vi "4155C Config I Stress v2.0.vi"(3 "Stress I - Drain/Gate":u32(ring)=1 items=["SMU1  ", "SMU2  ", "SMU3  ", "SMU4  ", "SMU5  ", "SMU6  "], 4 "Stress I - Source/Common":u32(ring) items=["SMU1  ", "SMU2  ", "SMU3  ", "SMU4  ", "SMU5  ", "SMU6  "], 5 "Display on/off":bool, 6 "error in (no error)":errorcluster, 7 "VDG compliance":dbl min=0.0 max=100000000000.0 format="%.15e", 8 "IDG":dbl min=0.0 max=100000000000.0 format="%.15e", 9 "VISA session":refnum<visa-resource-name>) -> (0 "error out":errorcluster, 2 "dup VISA resource name":refnum<visa-resource-name>)   [LabVIEW 2016]
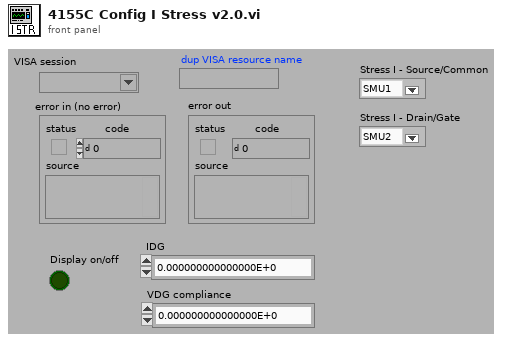
[diagram p1: front panel]
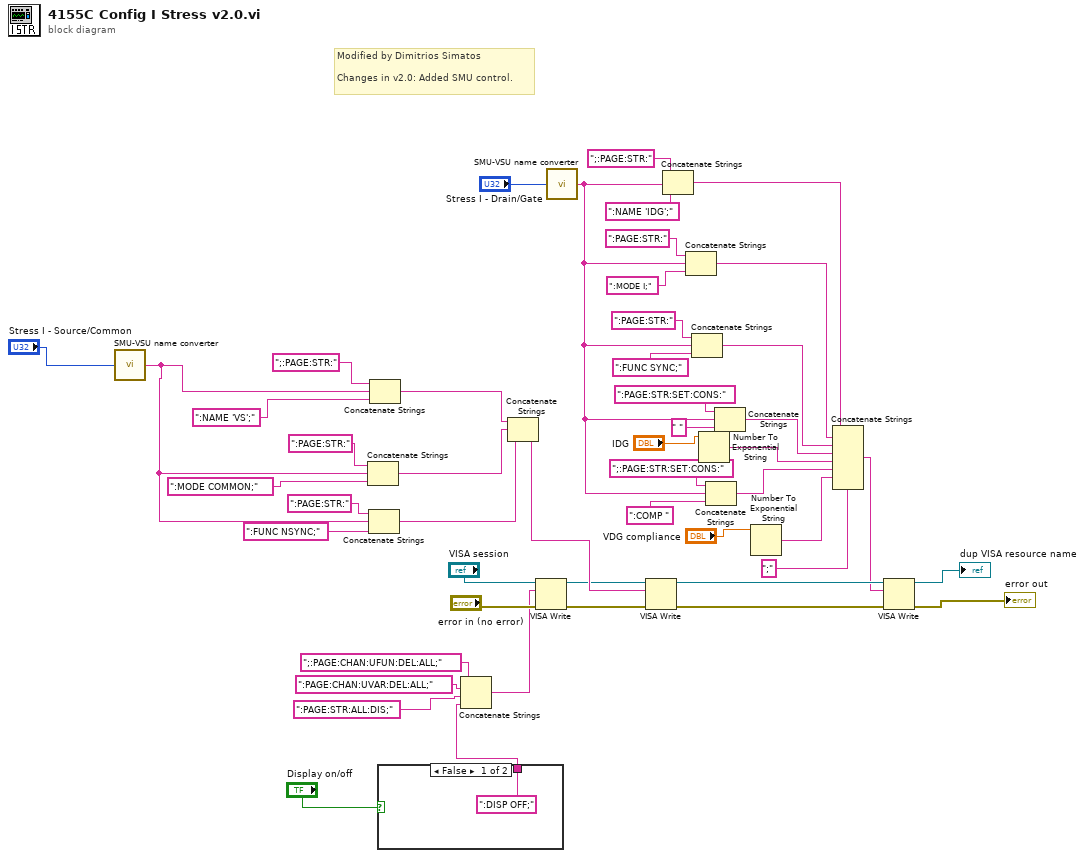
[diagram p0: block diagram]
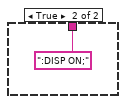
[diagram p2: hidden frame]
diagram:
  # "Modified by Dimitrios Simatos\n\nChanges in v2.0: Added SMU control."
  n1 = call "SMU-VSU name converter.vi"("unit to configure"="Stress I - Source/Common") -> ("SMU/VSU to be configured"=w23:string)
  n2 = Concatenate Strings(":PAGE:STR:", w23, ":MODE COMMON;") -> (w24:string)
  n3 = Concatenate Strings(":PAGE:STR:", w23, ":FUNC NSYNC;") -> (w22:string)
  n4 = Concatenate Strings(";:PAGE:STR:", w23, ":NAME 'VS';") -> (w28:string)
  n5 = case shown="False" "Display on/off" {
    tunnel: [":DISP OFF;" ("write buffer (\"\")") ":DISP ON;" ("write buffer (\"\")")] -> w43
    frame False {
    }
    frame True {
    }
  }
  n6 = Concatenate Strings(";:PAGE:CHAN:UFUN:DEL:ALL;", ":PAGE:CHAN:UVAR:DEL:ALL;", ":PAGE:STR:ALL:DIS;", w43) -> (w44:string)
  n7 = Concatenate Strings(w28, w24, w22) -> (w34:string)
  n8 = VISA Write(VISA resource name="VISA session", write buffer=w44, error in (no error)="error in (no error)") -> (VISA resource name out=w33:refnum<visa-resource-name>, error out=w32:errorcluster)  [unwired: 1 out]
  n9 = call "SMU-VSU name converter.vi"("unit to configure"="Stress I - Drain/Gate") -> ("SMU/VSU to be configured"=w2:string)
  n10 = VISA Write(VISA resource name=w33, write buffer=w34, error in (no error)=w32) -> (VISA resource name out=w49:refnum<visa-resource-name>, error out=w48:errorcluster)  [unwired: 1 out]
  n11 = Concatenate Strings(";:PAGE:STR:", w2, ":NAME 'IDG';") -> (w14:string)
  n12 = Concatenate Strings(":PAGE:STR:", w2, ":MODE I;") -> (w11:string)
  n13 = Concatenate Strings(":PAGE:STR:", w2, ":FUNC SYNC;") -> (w8:string)
  n14 = Number To Exponential String(number="IDG") -> (E-format string=w37:string)  [unwired: 3 in]
  n15 = Concatenate Strings(";:PAGE:STR:SET:CONS:", w2, ":COMP ") -> (w3:string)
  n16 = Concatenate Strings(":PAGE:STR:SET:CONS:", w2, " " ("string")) -> (w6:string)
  n17 = Number To Exponential String(number="VDG compliance") -> (E-format string=w35:string)  [unwired: 3 in]
  n18 = Concatenate Strings(w14, w11, w8, w6, w37, w3, w35, ";" ("Substring")) -> (w31:string)
  n19 = VISA Write(VISA resource name=w49, write buffer=w31, error in (no error)=w48) -> (VISA resource name out=→"dup VISA resource name":refnum<visa-resource-name>, error out=→"error out":errorcluster)  [unwired: 1 out]
